vi "_FPGA Read ADC.vi"(6 "error in":errorcluster, 8 "ADC Channel (64)":u8=64) -> (0 "error out":errorcluster, 1 "Running":bool, 2 "User Value":sgl, 3 "ADC Values":i32[](array[numeric]), 4 "In Range?":bool, 5 "Raw Reading":sgl)   [LabVIEW 2015]
uses:
  Type/_FPGA Indicator.ctl
  _RT Global.vi
  <vilib>/Utility/error.llb/Error Cluster From Error Code.vi
  <vilib>/rvi/errors/niLvFpgaAdjustHostInterfaceError.vi
  <vilib>/rvi/interface/nirviReadWriteControl/nirviReadWriteControl.xnode
  Type/FPGA Typedef.ctl
  FPGA Bitfiles/FPGA9607.lvbitx
  NiFpgaLv.dll
panel:
  out "Array":sgl[](array[numeric])
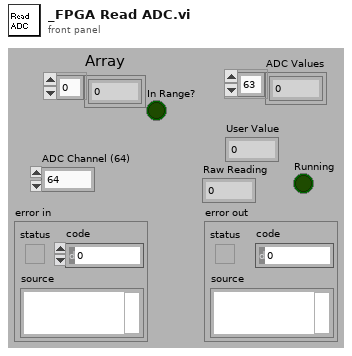
[diagram p1: front panel]
types:
  T1 = typedef "Semaphore RefNum" = refnum<k1>
  T2 = typedef "_FPGA Indicator.ctl" = enum16{"Done", "Ready", "Count Available", "SendSerial", "LED State"}
  T3 = typedef "FPGA Typedef.ctl" = refnum<k20>
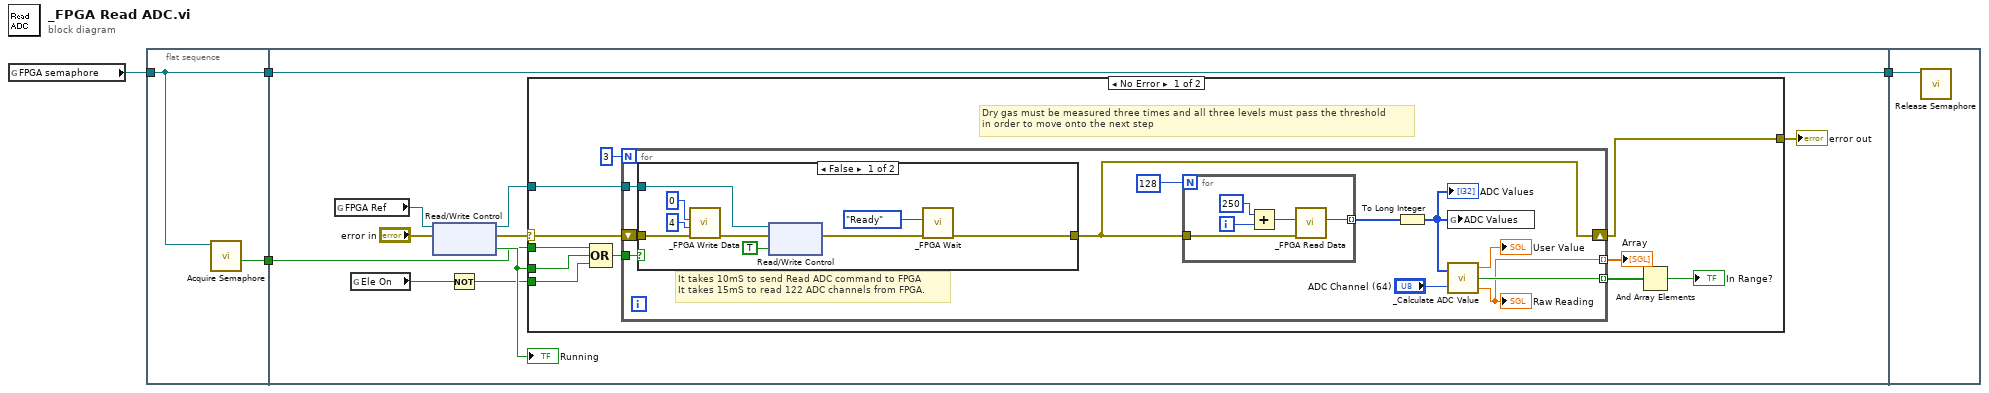
[diagram p0: block diagram]
diagram:
  n1 = global read "_RT Global.vi" "FPGA semaphore"() -> (w4:T1)
  n2 = flat-sequence {
    tunnel: w4 -> [w6]
    tunnel: [w6] -> w3
    tunnel: [w5] -> w2
    tunnel: w3 -> [w7]
    tunnel: [w7] -> w1
    tunnel: w2 -> [w9]
    tunnel: w1 -> [w55]
    frame #0 {
      n3 = call <vilib>:"Acquire Semaphore.vi"("semaphore"=w6) -> ("timed out"=w5:bool)  [unwired: 2 in, 4 out]
    }
    frame #1 {
      n4 = global read "_RT Global.vi" "FPGA Ref"() -> (w8:T3)
      n5 = global read "_RT Global.vi" "Ele On"() -> (w11:bool)
      n6 = xnode "Read/Write Control"("FPGA VI Reference In"=w8, "error in"="error in") -> ("FPGA VI Reference Out"=w14:T3, "error out"=w15:errorcluster, "Running"=w12:bool)
      "Running" <- w12
      n7 = Not(x=w11) -> (.not. x?=w10:bool)
      n8 = case shown="No Error" w15 {
        selector: w15 -> [w27 w54]
        tunnel: [w21 w54] -> w16
        tunnel: w14 -> [w26 _]
        tunnel: w12 -> [w25 _]
        tunnel: w10 -> [w23 _]
        tunnel: w9 -> [w22 _]
        frame No Error {
          # "Dry gas must be measured three times and all three levels must pass the threshold\nin order to move onto the next step"
          n9 = Compound Arithmetic op=OR(w22, w25, w23) -> (w24:bool)
          n10 = for {
            N: 3 -> [_]
            tunnel: w26 -> [w37]
            tunnel: w24 -> [w36]
            tunnel: [w35] -> w20 mode=indexing
            tunnel: [w34] -> w18 mode=indexing
            shift-right: [w28] -> w21
            shift-left: w27 -> [w38]
            # "It takes 10mS to send Read ADC command to FPGA\nIt takes 15mS to read 122 ADC channels from FPGA."
            n11 = case shown="False" w36 {
              tunnel: [w49 w53] -> w28
              tunnel: w38 -> [w51 w53]
              tunnel: w37 -> [w50 _]
              frame False {
                n12 = call "_FPGA Write Data.vi"("error in"=w51, "Data"=u32 4 ("Address"), "Address"=u16 0) -> ("error out"=w48:errorcluster)  [unwired: 3 in, 2 out]
                n13 = xnode "Read/Write Control"("FPGA VI Reference In"=w50, "error in"=w48, "Start"=TRUE) -> ("error out"=w52:errorcluster)  [unwired: 1 out]
                n14 = call "_FPGA Wait.vi"("error in"=w52, "Indicator"=_FPGA_Indicator."Ready") -> ("error out"=w49:errorcluster)  [unwired: 3 in, 2 out]
              }
              frame True {
              }
            }
            n15 = for {
              N: 128 -> [_]
              tunnel: [w40] -> w31 mode=indexing
              tunnel: w28 -> [w39]
              i -> [w41]
              n16 = Add(x=250, y=w41) -> (x+y=w42:i32)
              n17 = call "_FPGA Read Data.vi"("error in"=w39, "Address"=w42) -> ("Data"=w40:u32)  [unwired: 3 in, 2 out]
            }
            n18 = To Long Integer(number=w31) -> (32bit integer=w30:i32[])
            "ADC Values" <- w30
            n19 = global write "_RT Global.vi" "ADC Values"(w30) -> ()
            n20 = call "_Calculate ADC Value.vi"("ADC Values"=w30, "ADC Channel (64)"="ADC Channel (64)") -> ("User Value"=→"User Value":sgl, "In Range?"=w35:bool, "Raw Reading"=w34:sgl)
            "Raw Reading" <- w34
          }
          "Array" <- w18
          n21 = And Array Elements(Boolean array=w20) -> (logical AND=→"In Range?":bool)
        }
        frame Error {
        }
      }
      "error out" <- w16
    }
    frame #2 {
      n22 = call <vilib>:"Release Semaphore.vi"("semaphore"=w55) -> ()  [unwired: 1 in, 6 out]
    }
  }
